vi "stop.vi"(8 "error in (no error)":errorcluster, 11 "DAQ_DL091205Readers in":refnum<class "DAQ_DL091205Readers.lvclass">) -> (0 "error out":errorcluster, 3 "DAQ_DL091205Readers out":refnum<class "DAQ_DL091205Readers.lvclass">)   [LabVIEW 2010, in "DAQ_DL091205Readers.lvclass"]
uses:
  DAQ_DL091205Readers.lvclass
  DAQ_DL091205Readers.lvclass/DAQ_DL091205Readers.ctl
  SignalReader/GenericSignalReader/GenericSignalReader/GenericSignalReader.lvclass
  DAQ_DL090211Scaffold/DAQ_DL090211Scaffold/DAQ_DL090211Scaffold.lvclass
  common/classes/ErrorController/ErrorController/class_data.vi
  common/classes/ErrorController/ErrorController/ErrorController.lvclass
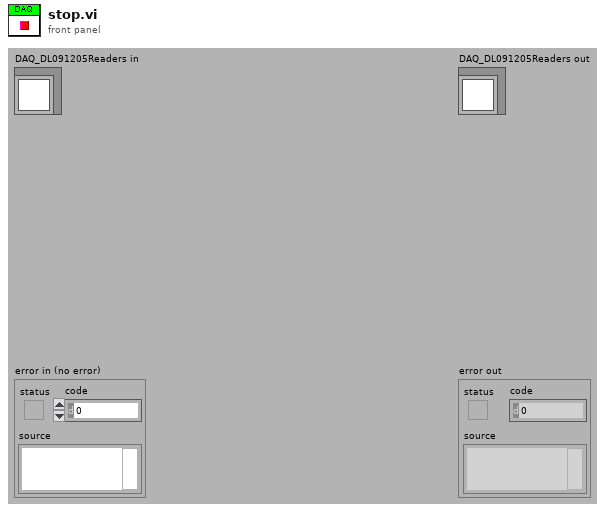
[diagram p1: front panel]
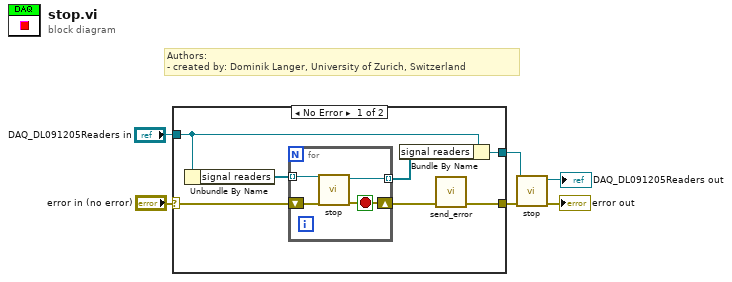
[diagram p0: block diagram]
diagram:
  # "Authors: \n- created by: Dominik Langer, University of Zurich, Switzerland"
  n1 = case shown="No Error" "error in (no error)" {
    selector: "error in (no error)" -> [w13 w19]
    tunnel: "DAQ_DL091205Readers in" -> [w10 w18]
    tunnel: [w8 w19] -> w4
    tunnel: [w9 w18] -> w3
    frame No Error {
      n2 = Unbundle By Name(w10) -> ("signal readers"=w12:refnum<class "GenericSignalReader.lvclass">[])
      n3 = for {
        tunnel: w12 -> [w16] mode=indexing
        tunnel: [w15] -> w11 mode=indexing
        shift-right: [w14] -> w7
        shift-left: w13 -> [w17]
        stop <- w14 stop-if-true
        n4 = call-dynamic "stop.vi"("error in (no error)"=w17, "GenericSignalReader in"=w16) -> ("error out"=w14:errorcluster, "GenericSignalReader out"=w15:refnum<class "GenericSignalReader.lvclass">)  [unwired: 8 in]
      }
      n5 = Bundle By Name(cluster=w10, "signal readers"=w11) -> (w9:refnum<class "DAQ_DL091205Readers.lvclass">)
      n6 = call "send_error.vi"("error in (no error)"=w7) -> ("error out"=w8:errorcluster)  [unwired: 10 in]
    }
    frame Error {
    }
  }
  n7 = call-parent "stop.vi"("error in (no error)"=w4, "DAQ_DL090211Scaffold in"=w3) -> ("error out"=→"error out":errorcluster, "DAQ_DL090211Scaffold out"=→"DAQ_DL091205Readers out":refnum<class "DAQ_DL091205Readers.lvclass">)  [unwired: 8 in]
